vi "FTP_USER.vi"(0 "connection ID":refnum<k5>, 1 "user":string, 2 "error out":errorcluster) -> (3 "connection ID out":refnum<k5>, 4 "reply string":string, 5 "Good Reply?":bool, 6 "error out 2":errorcluster)   [LabVIEW 2012]
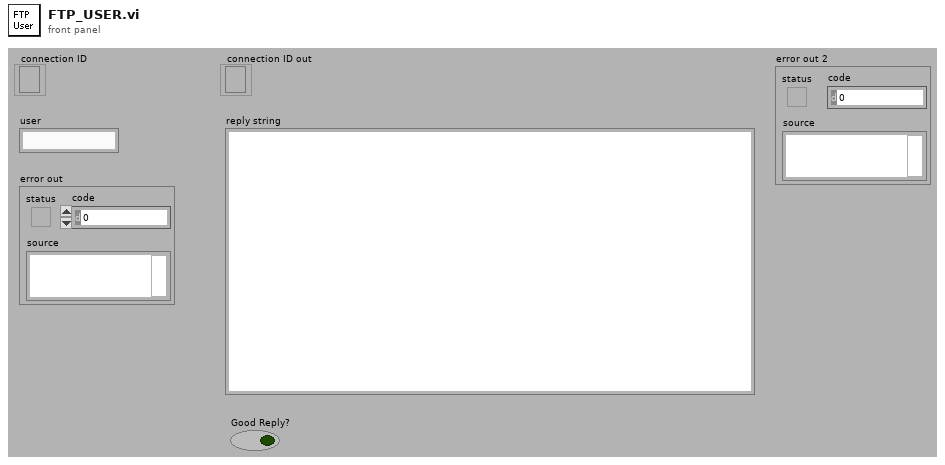
[diagram p1: front panel]
types:
  T1 = enum16{"unknown", "100 + Prelim", "200 + ", "300 + Intermed", "400 - Transient", "500 - Permanent"}
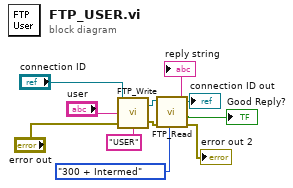
[diagram p0: block diagram]
diagram:
  n1 = call <userlib>:"FTP_Write.vi"("Cmd"="USER", "error in"="error out", "data"="user", "connection ID in"="connection ID") -> ("error out"=w2:errorcluster, "connection ID out"=w1:refnum<k5>)
  n2 = call <userlib>:"FTP_Read.vi"("error In"=w2, "expected class"=T1."300 + Intermed", "connection ID"=w1) -> ("error out"=→"error out 2":errorcluster, "Good Reply?"=→"Good Reply?":bool, "reply string"=→"reply string":string, "connection ID out"=→"connection ID out":refnum<k5>)  [unwired: 1 out]
